vi "Main.vi"() -> ()   [LabVIEW 2013]
uses:
  Dii.ctl
  <vilib>/Utility/xml.llb/Write to XML File(string).vi
panel:
  in  "Зберегти дані":bool
  out "Резезультат сортування":T1(array[cluster])
  in  "Exit":bool
  in  "Тестування датчиків тиску":T1(array[cluster])
  in  "Тиск (Р)":bool
  in  "Серійний №":bool
  in  "№ заказу":bool
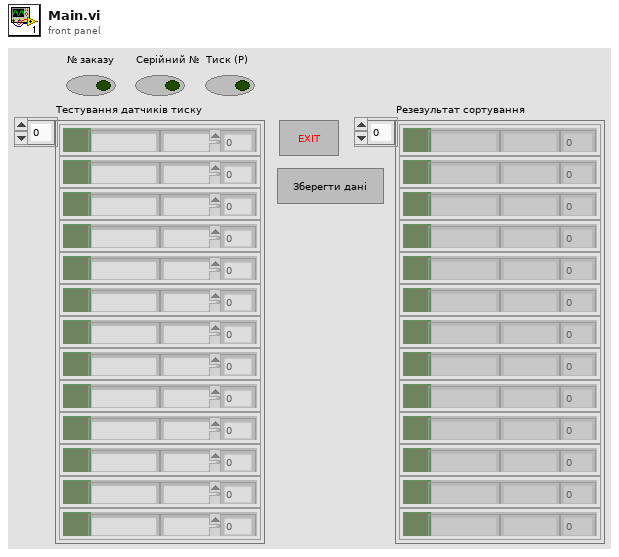
[diagram p1: front panel]
types:
  T1 = cluster{"ПН":bool, "№ заказу":string, "Серійний №":string, "Тиск (Р)":dbl}[]
  T2 = typedef "Dii.ctl" = enum16{"# Zak", "Ser #", "P", "Zapys", "Exit", "Onovlen"}
  T3 = cluster{"ПН":bool, "№ заказу":string, "Серійний №":string, "Тиск (Р)":dbl}
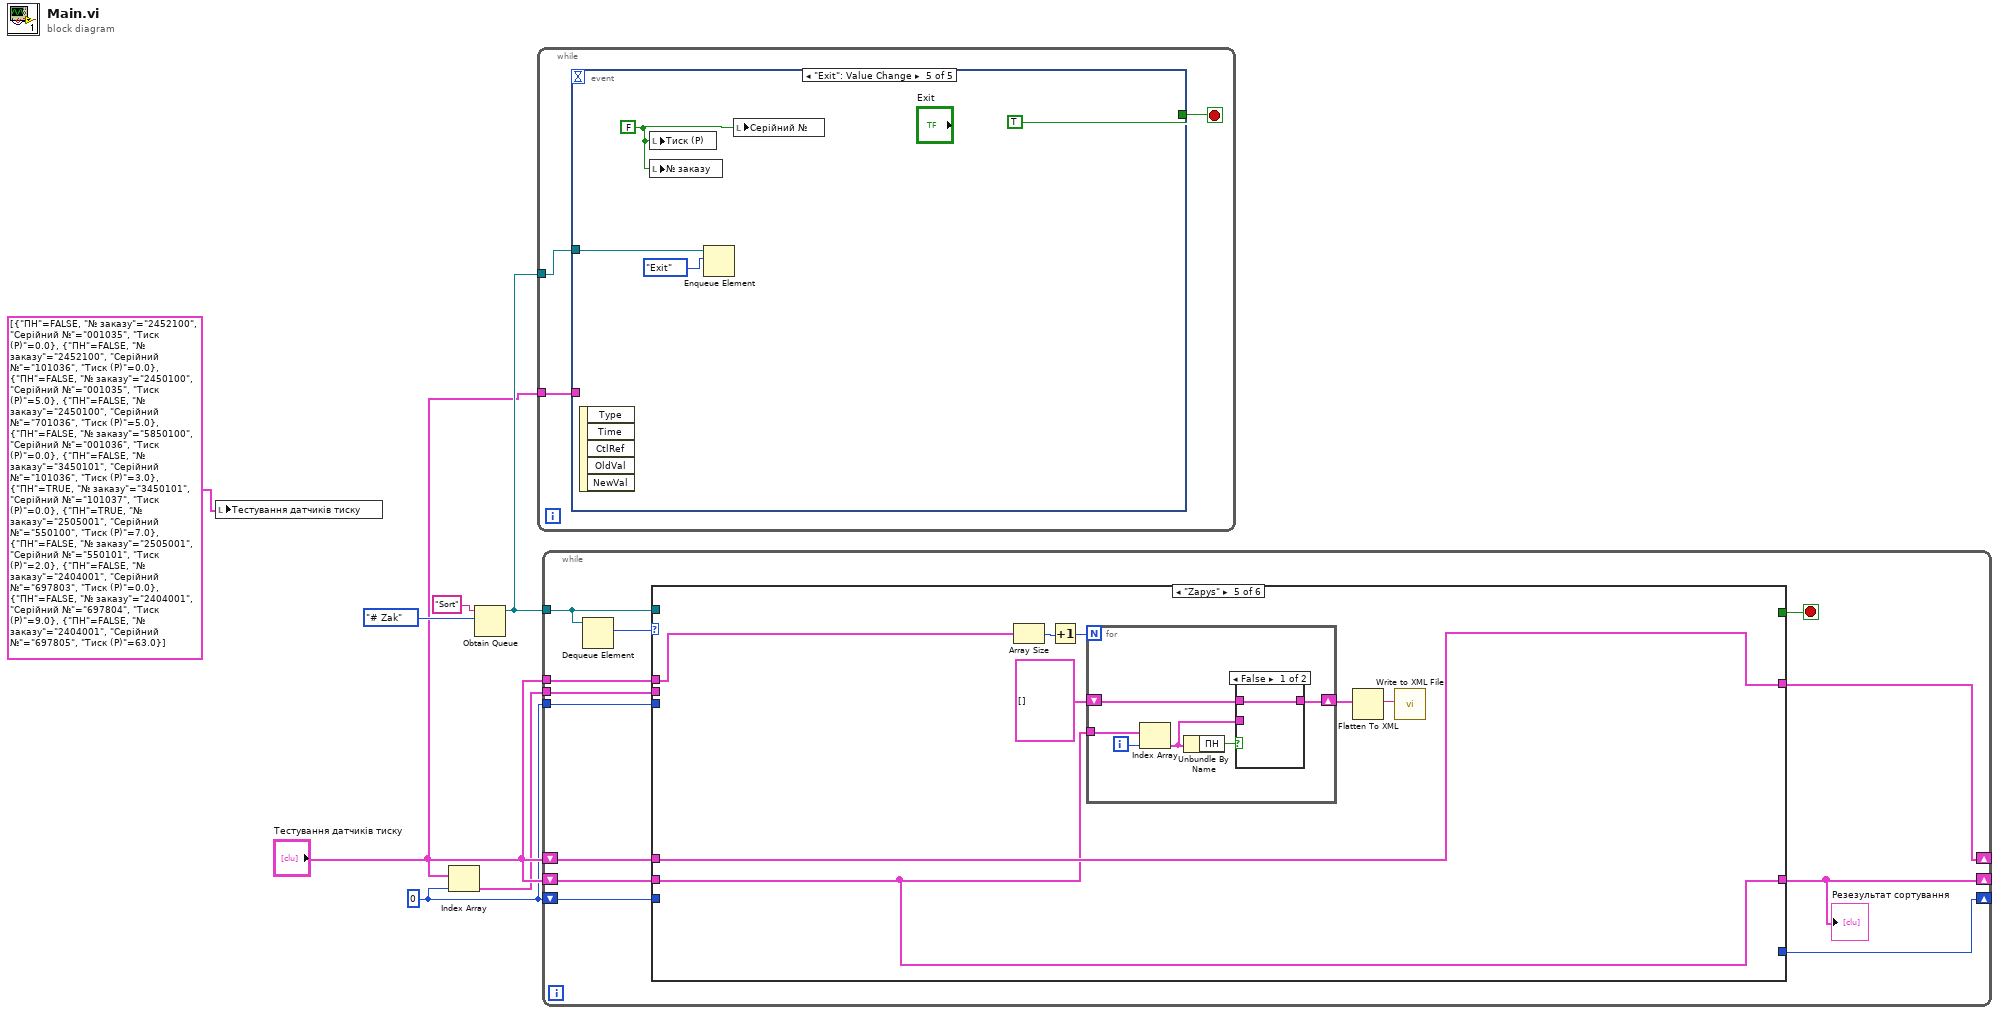
[diagram p0: block diagram]
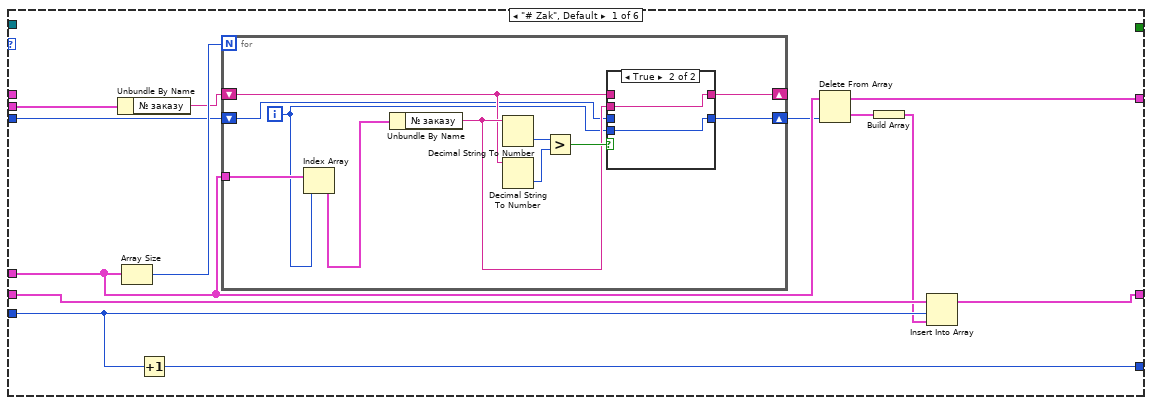
[diagram p2: hidden frame]
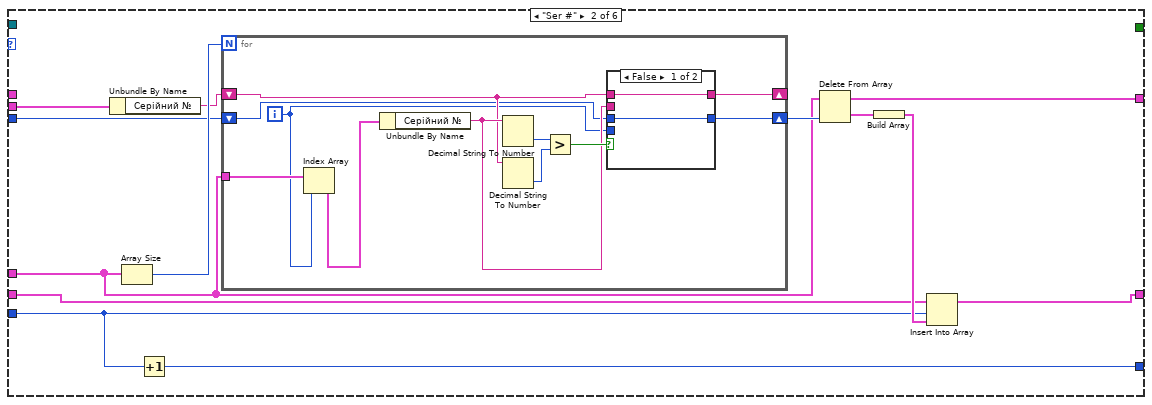
[diagram p4: hidden frame]
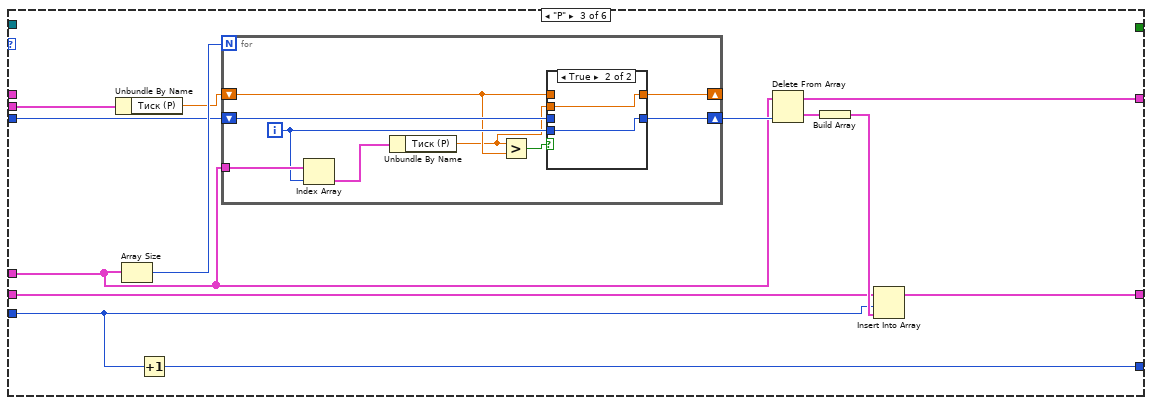
[diagram p6: hidden frame]
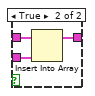
[diagram p9: hidden frame]
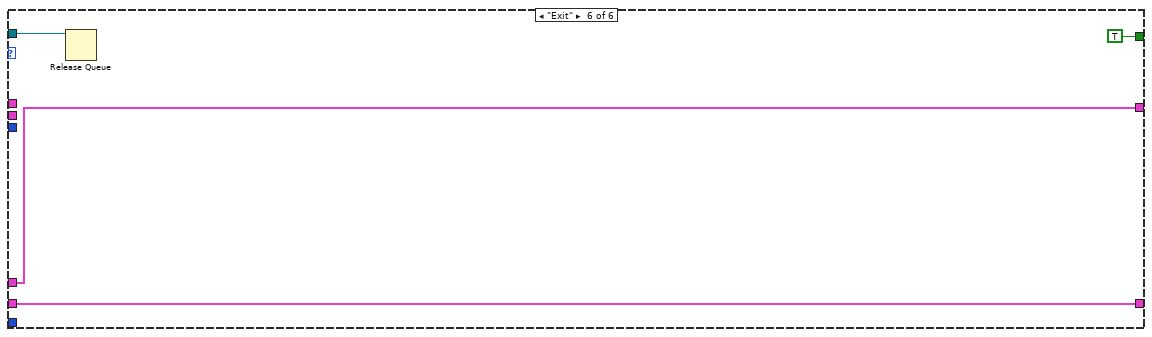
[diagram p10: hidden frame]
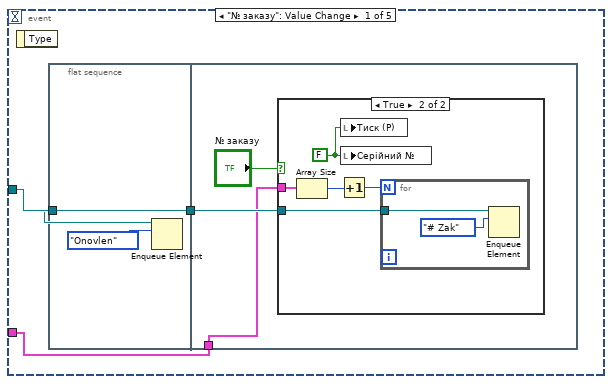
[diagram p11: hidden frame]
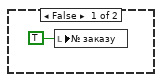
[diagram p12: hidden frame]
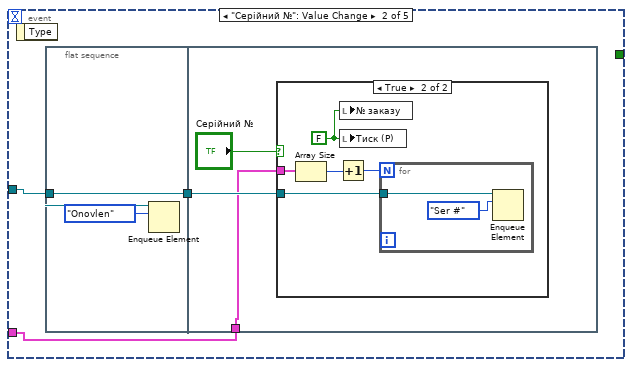
[diagram p13: hidden frame]
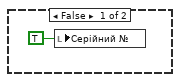
[diagram p14: hidden frame]
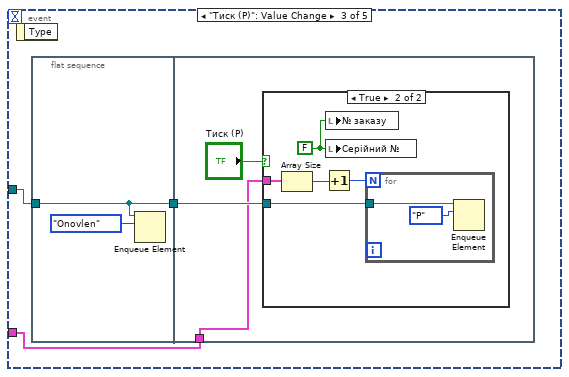
[diagram p15: hidden frame]
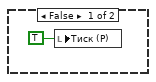
[diagram p16: hidden frame]
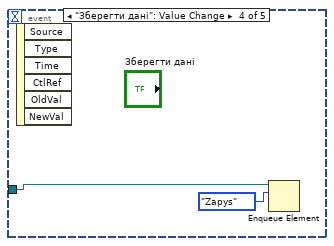
[diagram p17: hidden frame]
diagram:
  w2 = 0 ("index")
  n1 = local write "Тестування датчиків тиску"(T1 [{"ПН"=FALSE, "№ заказу"="2452100", "Серійний №"="001035", "Тиск (Р)"=0.0}, {"ПН"=FALSE, "№ заказу"="2452100", "Серійний №"="101036", "Тиск (Р)"=0.0}, {"ПН"=FALSE, "№ заказу"="2450100", "Серійний №"="001035", "Тиск (Р)"=5.0}, {"ПН"=FALSE, "№ заказу"="2450100", "Серійний №"="701036", "Тиск (Р)"=5.0}, {"ПН"=FALSE, "№ заказу"="5850100", "Серійний №"="001036", "Тиск (Р)"=0.0}, {"ПН"=FALSE, "№ заказу"="3450101", "Серійний №"="101036", "Тиск (Р)"=3.0}, {"ПН"=TRUE, "№ заказу"="3450101", "Серійний №"="101037", "Тиск (Р)"=0.0}, {"ПН"=TRUE, "№ заказу"="2505001", "Серійний №"="550100", "Тиск (Р)"=7.0}, {"ПН"=FALSE, "№ заказу"="2505001", "Серійний №"="550101", "Тиск (Р)"=2.0}, {"ПН"=FALSE, "№ заказу"="2404001", "Серійний №"="697803", "Тиск (Р)"=0.0}, {"ПН"=FALSE, "№ заказу"="2404001", "Серійний №"="697804", "Тиск (Р)"=9.0}, {"ПН"=FALSE, "№ заказу"="2404001", "Серійний №"="697805", "Тиск (Р)"=63.0}] ("Тестування датчиків тиску")) -> ()
  n2 = Index Array(array="Тестування датчиків тиску", index=w2) -> (element=w3:T3)
  n3 = Obtain Queue(name (unnamed)="Sort", element data type=Dii."# Zak" ("Enum")) -> (queue out=w5:refnum<queue>)  [unwired: 3 in, 2 out]
  n4 = while {
    tunnel: w5 -> [w10]
    tunnel: "Тестування датчиків тиску" -> [w8]
    stop <- w9 stop-if-true
    n5 = event shown="[4] \"Exit\": Value Change" {
      selector: _ -> [_ _ _ _ _]
      dyn-events: _ -> [_ _ _ _ _]
      timeout: _ -> [_ _ _ _ _]
      tunnel: w10 -> [w13 w29 w45 w59 w61]
      tunnel: [_ _ _ _ TRUE] -> w9
      tunnel: w8 -> [w11 w27 w43 _ _]
      event "№ заказу": Value Change {
        n6 = event-data() -> ()  [unwired: 1 in, 1 out]
        n7 = flat-sequence {
          tunnel: w13 -> [w14]
          tunnel: [w14] -> w12
          tunnel: w12 -> [w17]
          tunnel: w11 -> [w16]
          frame #0 {
            n8 = Enqueue Element(queue=w14, element=Dii."Onovlen" ("Enum")) -> ()  [unwired: 2 in, 3 out]
          }
          frame #1 {
            n9 = case shown="True" "№ заказу" {
              tunnel: w17 -> [_ w23]
              tunnel: w16 -> [_ w22]
              frame False {
                n10 = local write "№ заказу"(TRUE) -> ()
              }
              frame True {
                w24 = FALSE
                n11 = Array Size(array=w22) -> (size(s)=w21:i32)
                n12 = Increment(x=w21) -> (x+1=w20:i32)
                n13 = local write "Тиск (Р)"(w24) -> ()
                n14 = local write "Серійний №"(w24) -> ()
                n15 = for {
                  N: w20 -> [_]
                  tunnel: w23 -> [w25]
                  n16 = Enqueue Element(queue=w25, element=Dii."# Zak") -> ()  [unwired: 2 in, 3 out]
                }
              }
            }
          }
        }
      }
      event "Серійний №": Value Change {
        n17 = event-data() -> ()  [unwired: 1 in, 1 out]
        n18 = flat-sequence {
          tunnel: w29 -> [w30]
          tunnel: [w30] -> w28
          tunnel: w28 -> [w33]
          tunnel: w27 -> [w32]
          frame #0 {
            n19 = Enqueue Element(queue=w30, element=Dii."Onovlen" ("Enum")) -> ()  [unwired: 2 in, 3 out]
          }
          frame #1 {
            n20 = case shown="True" "Серійний №" {
              tunnel: w33 -> [_ w39]
              tunnel: w32 -> [_ w38]
              frame False {
                n21 = local write "Серійний №"(TRUE ("Серійний №")) -> ()
              }
              frame True {
                w40 = FALSE
                n22 = Array Size(array=w38) -> (size(s)=w37:i32)
                n23 = Increment(x=w37) -> (x+1=w36:i32)
                n24 = local write "№ заказу"(w40) -> ()
                n25 = local write "Тиск (Р)"(w40) -> ()
                n26 = for {
                  N: w36 -> [_]
                  tunnel: w39 -> [w41]
                  n27 = Enqueue Element(queue=w41, element=Dii."Ser #") -> ()  [unwired: 2 in, 3 out]
                }
              }
            }
          }
        }
      }
      event "Тиск (Р)": Value Change {
        n28 = event-data() -> ()  [unwired: 1 in, 1 out]
        n29 = flat-sequence {
          tunnel: w45 -> [w47]
          tunnel: [w47] -> w44
          tunnel: w44 -> [w50]
          tunnel: w43 -> [w48]
          frame #0 {
            n30 = Enqueue Element(queue=w47, element=Dii."Onovlen" ("Enum")) -> ()  [unwired: 2 in, 3 out]
          }
          frame #1 {
            n31 = case shown="True" "Тиск (Р)" {
              tunnel: w50 -> [_ w53]
              tunnel: w48 -> [_ w52]
              frame False {
                n32 = local write "Тиск (Р)"(TRUE) -> ()
              }
              frame True {
                w56 = FALSE
                n33 = Array Size(array=w52) -> (size(s)=w55:i32)
                n34 = Increment(x=w55) -> (x+1=w54:i32)
                n35 = local write "№ заказу"(w56) -> ()
                n36 = local write "Серійний №"(w56) -> ()
                n37 = for {
                  N: w54 -> [_]
                  tunnel: w53 -> [w57]
                  n38 = Enqueue Element(queue=w57, element=Dii."P") -> ()  [unwired: 2 in, 3 out]
                }
              }
            }
          }
        }
      }
      event "Зберегти дані": Value Change {
        n39 = event-data() -> ()  [unwired: 1 in, 6 out]
        n40 = Enqueue Element(queue=w59, element=Dii."Zapys") -> ()  [unwired: 2 in, 3 out]
      }
      event "Exit": Value Change {
        w63 = FALSE
        n41 = event-data() -> ()  [unwired: 1 in, 5 out]
        n42 = local write "Тиск (Р)"(w63) -> ()
        n43 = local write "№ заказу"(w63) -> ()
        n44 = Enqueue Element(queue=w61, element=Dii."Exit") -> ()  [unwired: 2 in, 3 out]
        n45 = local write "Серійний №"(w63) -> ()
      }
    }
  }
  n46 = while {
    tunnel: w5 -> [w67]
    shift-right: [w66] -> _
    shift-left: "Тестування датчиків тиску" -> [w74]
    shift-right: [w71] -> _
    shift-left: w2 -> [w73]
    shift-right: [w65] -> _
    shift-left: "Тестування датчиків тиску" -> [w72]
    tunnel: "Тестування датчиків тиску" -> [w70]
    tunnel: w2 -> [w69]
    tunnel: w3 -> [w68]
    stop <- w75 stop-if-true
    n47 = Dequeue Element(queue=w67) -> (element=w76:T2)  [unwired: 2 in, 3 out]
    n48 = case shown="\"Zapys\"" w76 {
      tunnel: [_ _ _ _ _ TRUE] -> w75
      tunnel: w74 -> [w87 w111 w139 _ w164 w178]
      tunnel: w73 -> [w89 w113 w141 _ _ _]
      tunnel: w72 -> [w86 w109 w137 _ w160 w179]
      tunnel: [w85 w112 w140 _ _ _] -> w71
      tunnel: [w84 w110 w138 w159 w164 w178] -> w66
      tunnel: [w83 w108 w136 w159 w160 w179] -> w65
      tunnel: w70 -> [_ _ _ w159 w165 _]
      tunnel: w67 -> [_ _ _ _ _ w180]
      tunnel: w68 -> [w78 w106 w134 _ _ _]
      tunnel: w69 -> [w79 w105 w133 _ _ _]
      frame "# Zak", Default {
        n49 = Unbundle By Name(w78) -> ("№ заказу"=w77:string)
        n50 = Array Size(array=w87) -> (size(s)=w88:i32)
        n51 = Increment(x=w89) -> (x+1=w85:i32)
        n52 = for {
          N: w88 -> [_]
          tunnel: w87 -> [w99]
          shift-right: [w94] -> _
          shift-left: w77 -> [w93]
          shift-right: [w92] -> w82
          shift-left: w79 -> [w90]
          i -> [w91]
          n53 = Index Array(array=w99, index=w91) -> (element=w100:T3)
          n54 = Unbundle By Name(w100) -> ("№ заказу"=w95:string)
          n55 = Decimal String To Number(string=w95) -> (number=w98:i32)  [unwired: 2 in, 1 out]
          n56 = Decimal String To Number(string=w93) -> (number=w97:i32)  [unwired: 2 in, 1 out]
          n57 = Greater?(x=w98, y=w97) -> (0:w96:bool)
          n58 = case shown="True" w96 {
            tunnel: [w102 w104] -> w94
            tunnel: w95 -> [_ w104]
            tunnel: w93 -> [w102 _]
            tunnel: [w101 w103] -> w92
            tunnel: w91 -> [_ w103]
            tunnel: w90 -> [w101 _]
            frame False {
            }
            frame True {
            }
          }
        }
        n59 = Delete From Array(array=w87, index=w82) -> (deleted portion=w81:T3, array with subset deleted=w84:T1)  [unwired: 1 in]
        n60 = Build Array(w81) -> (w80:T1)
        n61 = Insert Into Array(array=w86, index=w89, new element=w80) -> (w83:T1)
      }
      frame "Ser #" {
        n62 = Unbundle By Name(w106) -> ("Серійний №"=w107:string)
        n63 = Array Size(array=w111) -> (size(s)=w117:i32)
        n64 = Increment(x=w113) -> (x+1=w112:i32)
        n65 = for {
          N: w117 -> [_]
          tunnel: w111 -> [w127]
          shift-right: [w122] -> _
          shift-left: w107 -> [w121]
          shift-right: [w120] -> w116
          shift-left: w105 -> [w118]
          i -> [w119]
          n66 = Index Array(array=w127, index=w119) -> (element=w128:T3)
          n67 = Unbundle By Name(w128) -> ("Серійний №"=w123:string)
          n68 = Decimal String To Number(string=w123) -> (number=w126:i32)  [unwired: 2 in, 1 out]
          n69 = Decimal String To Number(string=w121) -> (number=w125:i32)  [unwired: 2 in, 1 out]
          n70 = Greater?(x=w126, y=w125) -> (0:w124:bool)
          n71 = case shown="False" w124 {
            tunnel: [w130 w132] -> w122
            tunnel: w123 -> [_ w132]
            tunnel: w121 -> [w130 _]
            tunnel: [w129 w131] -> w120
            tunnel: w119 -> [_ w131]
            tunnel: w118 -> [w129 _]
            frame False {
            }
            frame True {
            }
          }
        }
        n72 = Delete From Array(array=w111, index=w116) -> (deleted portion=w115:T3, array with subset deleted=w110:T1)  [unwired: 1 in]
        n73 = Build Array(w115) -> (w114:T1)
        n74 = Insert Into Array(array=w109, index=w113, new element=w114) -> (w108:T1)
      }
      frame "P" {
        n75 = Unbundle By Name(w134) -> ("Тиск (Р)"=w135:dbl)
        n76 = Array Size(array=w139) -> (size(s)=w145:i32)
        n77 = Increment(x=w141) -> (x+1=w140:i32)
        n78 = for {
          N: w145 -> [_]
          tunnel: w139 -> [w153]
          shift-right: [w151] -> _
          shift-left: w135 -> [w147]
          shift-right: [w150] -> w144
          shift-left: w133 -> [w148]
          i -> [w149]
          n79 = Index Array(array=w153, index=w149) -> (element=w154:T3)
          n80 = Unbundle By Name(w154) -> ("Тиск (Р)"=w146:dbl)
          n81 = Greater?(x=w146, y=w147) -> (0:w152:bool)
          n82 = case shown="True" w152 {
            tunnel: [w156 w158] -> w151
            tunnel: w146 -> [_ w158]
            tunnel: w147 -> [w156 _]
            tunnel: [w155 w157] -> w150
            tunnel: w149 -> [_ w157]
            tunnel: w148 -> [w155 _]
            frame False {
            }
            frame True {
            }
          }
        }
        n83 = Delete From Array(array=w139, index=w144) -> (deleted portion=w143:T3, array with subset deleted=w138:T1)  [unwired: 1 in]
        n84 = Build Array(w143) -> (w142:T1)
        n85 = Insert Into Array(array=w137, index=w141, new element=w142) -> (w136:T1)
      }
      frame "Onovlen" {
      }
      frame "Zapys" {
        n86 = Array Size(array=w165) -> (size(s)=w167:i32)
        n87 = Increment(x=w167) -> (x+1=w166:i32)
        n88 = for {
          N: w166 -> [_]
          tunnel: w160 -> [w172]
          shift-right: [w168] -> w162
          shift-left: T1 [] -> [w169]
          i -> [w171]
          n89 = Index Array(array=w172, index=w171) -> (element=w170:T3)
          n90 = Unbundle By Name(w170) -> ("ПН"=w173:bool)
          n91 = case shown="False" w173 {
            tunnel: w170 -> [_ w177]
            tunnel: w169 -> [w174 w176]
            tunnel: [w174 w175] -> w168
            frame False {
            }
            frame True {
              n92 = Insert Into Array(array=w176, new element=w177) -> (w175:T1)  [unwired: 1 in]
            }
          }
        }
        n93 = Flatten To XML(anything=w162) -> (xml string=w163:string)
        n94 = call-poly <vilib>:"Write to XML File.vi"("XML Input"=w163) -> ()  [unwired: 8 in, 3 out]
      }
      frame "Exit" {
        n95 = Release Queue(queue=w180) -> ()  [unwired: 2 in, 3 out]
      }
    }
    "Резезультат сортування" <- w65
  }
